vi "Alpha 1.vi"() -> ()   [LabVIEW 2011]
panel:
  out "Path to Image":path
  out "2D Picture":picture
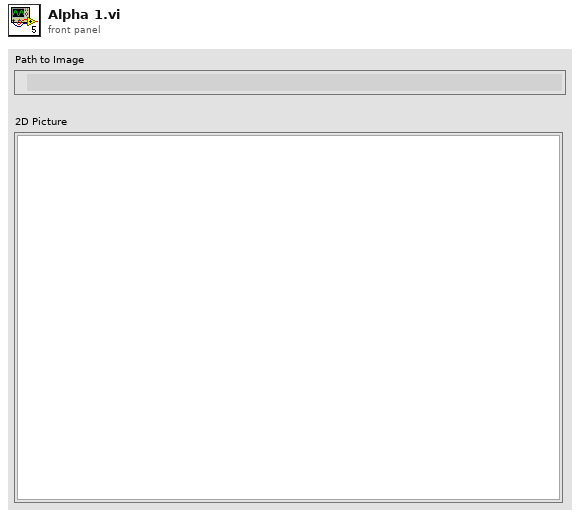
[diagram p1: front panel]
types:
  T1 = typedef "imagedata.ctl" = cluster{"image type":i32, "image depth":i32, "image":u8[], "mask":u8[], "colors":u32[], "Rectangle":cluster{"left":i16, "top":i16, "right":i16, "bottom":i16}}
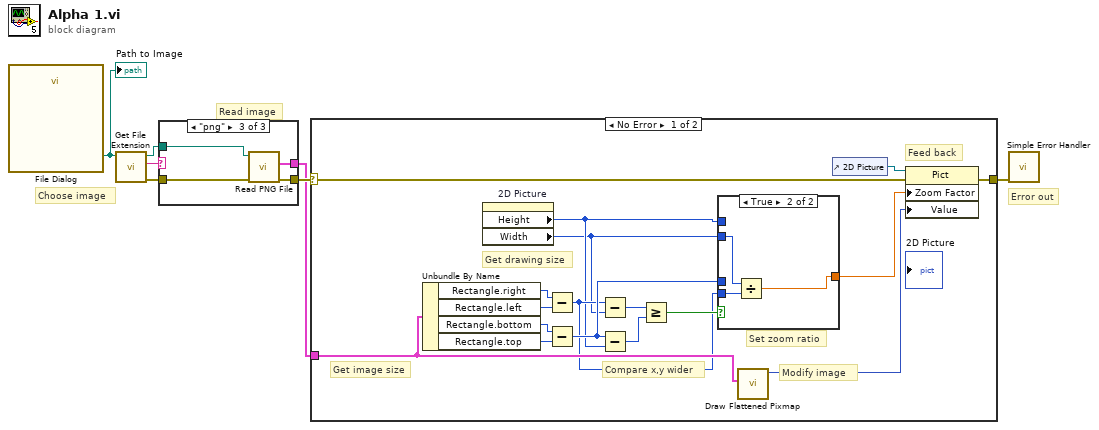
[diagram p0: block diagram]
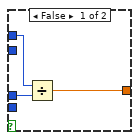
[diagram p2: hidden frame]
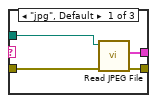
[diagram p4: hidden frame]
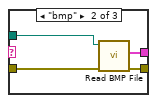
[diagram p5: hidden frame]
diagram:
  # "Choose image"
  # "Error out"
  # "Read image"
  n1 = call "File Dialog"() -> ("selected path"=w1:path)  [unwired: 12 in, 3 out]
  "Path to Image" <- w1
  n2 = call <vilib>:"Get File Extension.vi"("file"=w1) -> ("error out"=w3:errorcluster, "lowercase file extension"=w7:string, "dup file"=w2:path)  [unwired: 7 in, 1 out]
  n3 = case shown="\"png\"" w7 {
    tunnel: w2 -> [w11 w15 w19]
    tunnel: [w10 w14 w18] -> w5
    tunnel: [w9 w13 w17] -> w4
    tunnel: w3 -> [w8 w12 w16]
    frame "jpg", Default {
      n4 = call <vilib>:"Read JPEG File.vi"("error in (no error)"=w8, "path to JPEG file"=w11) -> ("error out"=w10:errorcluster, "image data"=w9:T1)  [unwired: 7 in, 1 out]
    }
    frame "bmp" {
      n5 = call <vilib>:"Read BMP File.vi"("error in (no error)"=w12, "path to BMP file"=w15) -> ("error out"=w14:errorcluster, "image data"=w13:T1)  [unwired: 7 in, 1 out]
    }
    frame "png" {
      n6 = call <vilib>:"Read PNG File.vi"("error in (no error)"=w16, "path to PNG file"=w19) -> ("error out"=w18:errorcluster, "image data"=w17:T1)  [unwired: 7 in, 1 out]
    }
  }
  n7 = case shown="No Error" w5 {
    selector: w5 -> [w31 w43]
    tunnel: w4 -> [w32 _]
    tunnel: [w29 w43] -> w6
    frame No Error {
      # "Modify image"
      # "Feed back"
      # "Set zoom ratio"
      # "Compare x,y wider"
      # "Get drawing size"
      # "Get image size"
      n8 = Unbundle By Name(w32) -> ("Rectangle.right"=w36:i16, "Rectangle.left"=w35:i16, "Rectangle.bottom"=w34:i16, "Rectangle.top"=w33:i16)
      n9 = property on="2D Picture" class="Pict"() -> ("Height"=w23:u32, "Width"=w22:u32)  [unwired: 2 in, 2 out]
      n10 = Subtract(x=w36, y=w35) -> (x-y=w24:i16)
      n11 = Subtract(x=w34, y=w33) -> (x-y=w25:i16)
      n12 = Subtract(x=w24, y=w22) -> (x-y=w28:u32)
      n13 = Subtract(x=w25, y=w23) -> (x-y=w27:u32)
      n14 = Greater Or Equal?(x=w28, y=w27) -> (x >= y?=w26:bool)
      n15 = case shown="True" w26 {
        tunnel: w23 -> [w39 _]
        tunnel: w25 -> [w38 _]
        tunnel: [w37 w42] -> w21
        tunnel: w22 -> [_ w41]
        tunnel: w24 -> [_ w40]
        frame False {
          n16 = Divide(x=w39, y=w38) -> (x/y=w37:dbl)
        }
        frame True {
          n17 = Divide(x=w41, y=w40) -> (x/y=w42:dbl)
        }
      }
      n18 = call <vilib>:"Draw Flattened Pixmap.vi"("image data"=w32) -> ("new picture"=w30:picture)  [unwired: 8 in]
      n19 = control-ref of="2D Picture"() -> (w20:refnum<vi>)
      n20 = property on="Property Node" class="Pict"(reference=w20, error in=w31, "Zoom Factor"=w21, "Value"=w30) -> (error out=w29:errorcluster)  [unwired: 1 out]
    }
    frame Error {
    }
  }
  n21 = call <vilib>:"Simple Error Handler.vi"("error in (no error)"=w6) -> ()  [unwired: 4 in, 5 out]
